vi "tm422_timelapse.vi"() -> ()   [LabVIEW 2011]
panel:
  in  "Interval (ms)":u32=500
  out "Timestamp":dbl
  out "DCAM Version":string
  out "Library Version":string
  out "Image":u16[][](graph)
  in  "Quit":bool
  out "Error Out":errorcluster {"code" format="%.0x"}
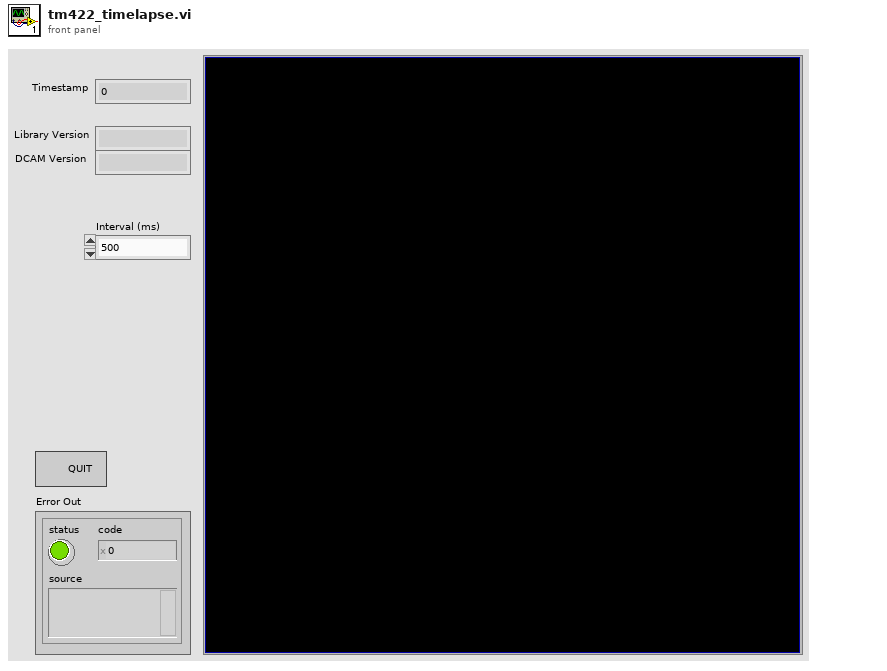
[diagram p1: front panel]
types:
  T1 = cluster{"Capture Library":string, "DCAM-API":string}
  T2 = cluster{"Mode":u32, "Polarity":u32, "Times":u32, "Delay":dbl}
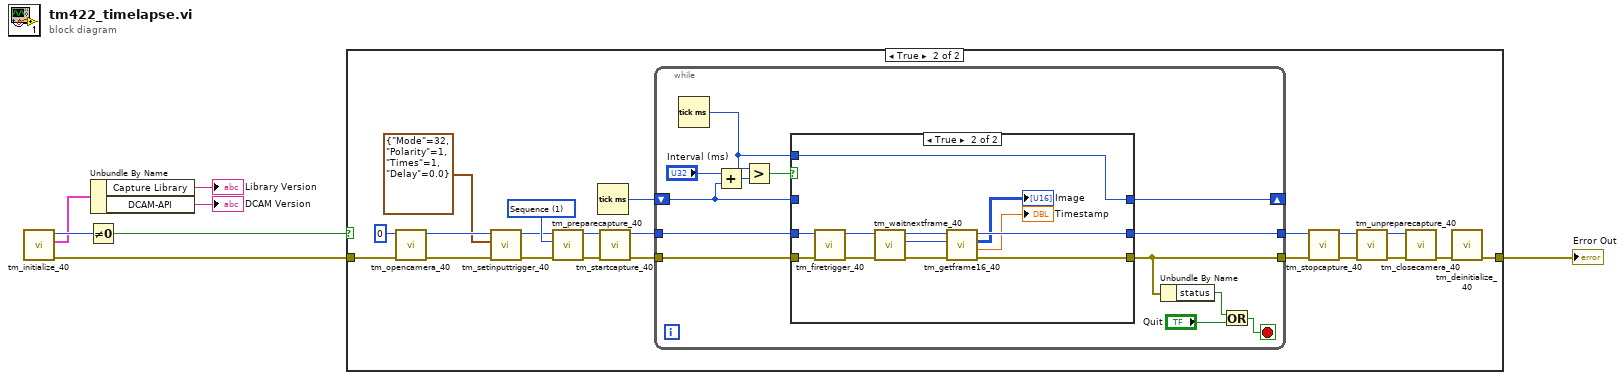
[diagram p0: block diagram]
diagram:
  n1 = call <userlib>:"tm_initialize_40.vi"() -> ("error out"=w4:errorcluster, "Version Info"=w3:T1, "Number Of Cameras"=w5:u32)  [unwired: 8 in, 1 out]
  n2 = Not Equal To 0?(x=w5) -> (x != 0?=w7:bool)
  n3 = Unbundle By Name(w3) -> ("Capture Library"=→"Library Version":string, "DCAM-API"=→"DCAM Version":string)
  n4 = case shown="True" w7 {
    tunnel: w4 -> [w8 w29]
    tunnel: [w8 w26] -> w6
    frame False {
    }
    frame True {
      w17 = 1 items=["Snap", "Sequence"] ("Capture mode")
      n5 = call <userlib>:"tm_opencamera_40.vi"("error in (no error)"=w29, "Camera Index"=u32 0) -> ("error out"=w10:errorcluster, "Handle out"=w11:u32)  [unwired: 7 in, 1 out]
      n6 = call <userlib>:"tm_setinputtrigger_40.vi"("error in (no error)"=w10, "Parameters"=T2 {"Mode"=32, "Polarity"=1, "Times"=1, "Delay"=0.0}, "Handle in"=w11) -> ("error out"=w13:errorcluster, "Handle out"=w12:u32)  [unwired: 7 in]
      n7 = call <userlib>:"tm_preparecapture_40.vi"("error in (no error)"=w13, "Capture mode"=w17, "Handle in"=w12) -> ("error out"=w15:errorcluster, "Handle out"=w16:u32)  [unwired: 5 in, 2 out]
      n8 = Tick Count (ms)() -> (millisecond timer value=w14:u32)
      n9 = call <userlib>:"tm_startcapture_40.vi"("error in (no error)"=w15, "Handle in"=w16) -> ("error out"=w18:errorcluster, "Handle out"=w19:u32)  [unwired: 8 in]
      n10 = while {
        tunnel: [w35] -> w22
        tunnel: [w36] -> w23
        tunnel: w19 -> [w32]
        tunnel: w18 -> [w31]
        shift-right: [w34] -> _
        shift-left: w14 -> [w37]
        stop <- w30 stop-if-true
        n11 = Tick Count (ms)() -> (millisecond timer value=w38:u32)
        n12 = Add(x="Interval (ms)", y=w37) -> (x+y=w40:u32)
        n13 = Greater?(x=w38, y=w40) -> (0:w39:bool)
        n14 = case shown="True" w39 {
          tunnel: w32 -> [w45 w46]
          tunnel: w31 -> [w44 w49]
          tunnel: w37 -> [w43 _]
          tunnel: w38 -> [_ w57]
          tunnel: [w45 w55] -> w35
          tunnel: [w44 w56] -> w36
          tunnel: [w43 w57] -> w34
          frame False {
          }
          frame True {
            n15 = call <userlib>:"tm_firetrigger_40.vi"("error in (no error)"=w49, "Handle in"=w46) -> ("error out"=w48:errorcluster, "Handle out"=w47:u32)  [unwired: 8 in]
            n16 = call <userlib>:"tm_waitnextframe_40.vi"("error in (no error)"=w48, "Handle in"=w47) -> ("error out"=w52:errorcluster, "Frame Index"=w50:i32, "Handle out"=w51:u32)  [unwired: 6 in, 1 out]
            n17 = call <userlib>:"tm_getframe16_40.vi"("error in (no error)"=w52, "Frame Index"=w50, "Handle in"=w51) -> ("error out"=w56:errorcluster, "Timestamp"=→"Timestamp":dbl, "Data"=→"Image":u16[][], "Handle out"=w55:u32)  [unwired: 5 in]
          }
        }
        n18 = Unbundle By Name(w36) -> ("status"=w42:bool)
        n19 = Or(x=w42, y="Quit") -> (x .or. y?=w30:bool)
      }
      n20 = call <userlib>:"tm_stopcapture_40.vi"("error in (no error)"=w23, "Handle in"=w22) -> ("error out"=w20:errorcluster, "Handle out"=w21:u32)  [unwired: 8 in]
      n21 = call <userlib>:"tm_unpreparecapture_40.vi"("error in (no error)"=w20, "Handle in"=w21) -> ("error out"=w25:errorcluster, "Handle out"=w24:u32)  [unwired: 8 in]
      n22 = call <userlib>:"tm_closecamera_40.vi"("error in (no error)"=w25, "Handle in"=w24) -> ("error out"=w27:errorcluster)  [unwired: 9 in]
      n23 = call <userlib>:"tm_deinitialize_40.vi"("error in (no error)"=w27) -> ("error out"=w26:errorcluster)  [unwired: 10 in]
    }
  }
  "Error Out" <- w6
